vi "Calibrate Ohms.vi"(5 "Device Name":string, 8 "error in (no error)":errorcluster, 9 "nDelayValue":i32, 10 "nScale":i32, 11 "Resistance":T1) -> (0 "error out":errorcluster, 3 "Return Code":i32)   [LabVIEW 2015]
doc: "This vi will write to the DAQ to set the relays for the selected resitance and then executes the ZeroCalibrateM5Ohms or the SpanCalibrateM5Ohms DLL call to calibrate the UUT"
uses:
  DAQ/Resistances.ctl
  DAQ/Relay Modes.ctl
  DAQ/Channels_v2.ctl
panel:
  # "4.1 SpanCalibrateM5Ohms 40 Ohm Zero NonZero\n4.2 SpanCalibrateM5Ohms 400 Ohm Zero NonZero\n4.3 SpanCalibrateM5Ohms 4K Ohm Zero NonZero\n4.4 SpanCalibrateM5Ohms 40K Ohm Zero NonZero\n4.5 SpanCalibrateM5Ohms 400K Ohm Zero NonZero\n4.6 SpanCalibrateM5Ohms 4 Meg Ohm Zero NonZero"
  # "`"
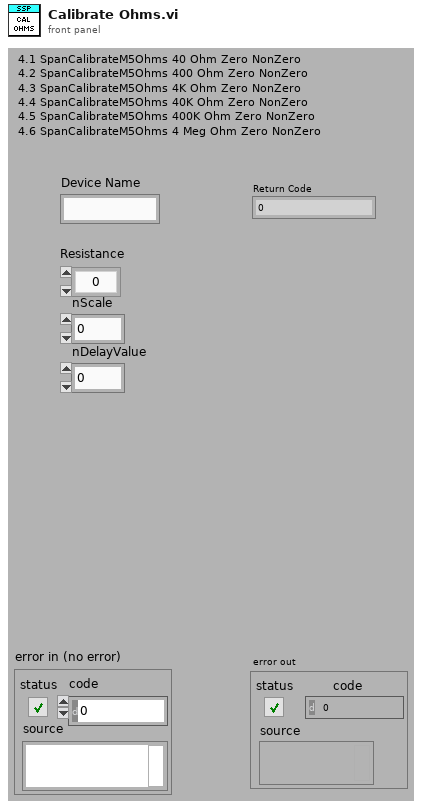
[diagram p1: front panel]
types:
  T1 = typedef "Resistances.ctl" = enum16{"0", "20", "40", "200", "400", "2k", "4K", "20k", "40K", "200k", "400K", "2M", "4M"}
  T2 = typedef "Channels_v2.ctl" = enum16{"All Off", "Channel 4", "Channel 3", "4,3", "Channel 2", "4,2", "3,2", "4,3,2,", "Channel 1", "4,1", "3,1", "4,3,1", "2,1", "4,2,1", "3,2,1", "All On"}
  T3 = typedef "Relay Modes.ctl" = enum16{"All Off", "Short", "Ohms", "Fluke", "Daq AO 0"}
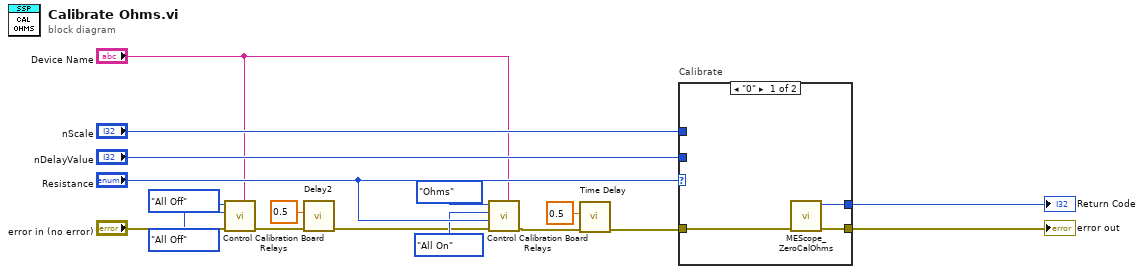
[diagram p0: block diagram]
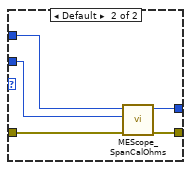
[diagram p2: hidden frame]
diagram:
  n1 = call "Control Calibration Board Relays.vi"("Device Name"="Device Name", "error in"="error in (no error)", "Channels"=Channels_v2."All Off", "Mode"=Relay_Modes."All Off") -> ("error out"=w2:errorcluster)  [unwired: 7 in]
  n2 = call "Delay2"("error in (no error)"=w2, "Delay Time (s)"=0.5) -> ("error out"=w1:errorcluster)  [unwired: 9 in]
  n3 = call "Control Calibration Board Relays.vi"("Device Name"="Device Name", "error in"=w1, "Resistance"="Resistance", "Channels"=Channels_v2."All On", "Mode"=Relay_Modes."Ohms") -> ("error out"=w14:errorcluster)  [unwired: 6 in]
  n4 = call "Time Delay"("error in (no error)"=w14, "Delay Time (s)"=0.5) -> ("error out"=w13:errorcluster)  [unwired: 9 in]
  n5 = case "Calibrate" shown="\"0\"" "Resistance" {
    tunnel: [w18 w25] -> w10
    tunnel: w13 -> [w20 w24]
    tunnel: [w19 w23] -> w11
    tunnel: "nScale" -> [_ w22]
    tunnel: "nDelayValue" -> [_ w21]
    frame "0" {
      n6 = call "MEScope_ZeroCalOhms.vi"("error in"=w20) -> ("error out"=w19:errorcluster, "Return Code"=w18:i32)  [unwired: 9 in]
    }
    frame Default {
      n7 = call "MEScope_SpanCalOhms.vi"("error in (no error)"=w24, "nDelayValue"=w21, "nScale"=w22) -> ("error out"=w23:errorcluster, "Return Code"=w25:i32)  [unwired: 7 in]
    }
  }
  "error out" <- w11
  "Return Code" <- w10
